vi "Create Typedef.vi"(6 "Location (0,0)":T1, 7 "Typedef Path":path, 8 "error in (no error)":errorcluster, 9 "Label":string, 11 "Owner in":refnum<vi>) -> (0 "error out":errorcluster, 2 "Typedef Control":refnum<vi>)   [LabVIEW 2020, in "LV-Protoc.lvlib"]
uses:
  LV-Protoc.lvlib
  <vilib>/Utility/miscctls.llb/LVPointTypeDef.ctl
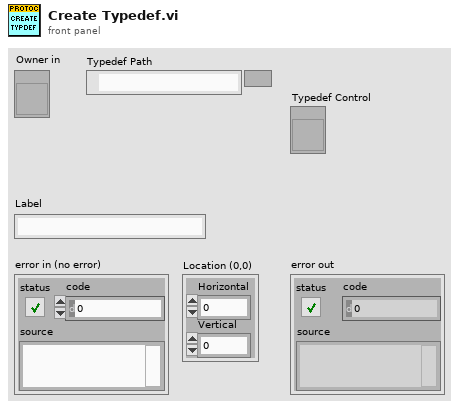
[diagram p1: front panel]
types:
  T1 = typedef "LVPointTypeDef.ctl" = cluster{"Horizontal":i16, "Vertical":i16}
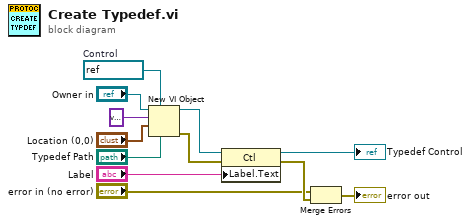
[diagram p0: block diagram]
diagram:
  w12 = refnum<vi> refnum  # Control
  n1 = New VI Object(vi object class=w12, owner refnum="Owner in", style=variant, position/next to="Location (0,0)", 6:"Typedef Path") -> (object refnum=w11:refnum<vi>, 0:w10:errorcluster)  [unwired: 3 in]
  n2 = property class="Ctl"(reference=w11, error in=w10, "Label.Text"="Label") -> (reference out=→"Typedef Control":refnum<vi>, error out=w6:errorcluster)
  n3 = Merge Errors("error in (no error)", w6) -> (→"error out":errorcluster)
